vi "BaudDetect-Make Success Info.vi"(10 "Normal":bool, 11 "list":refnum<vi>) -> (3 "Info":string)   [LabVIEW 2011]
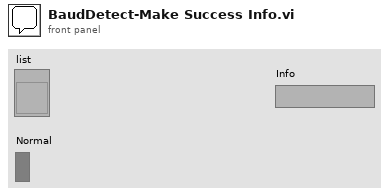
[diagram p1: front panel]
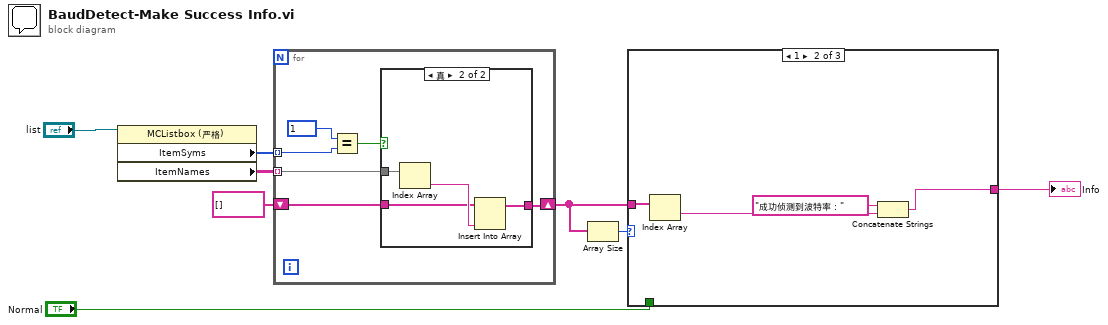
[diagram p0: block diagram]
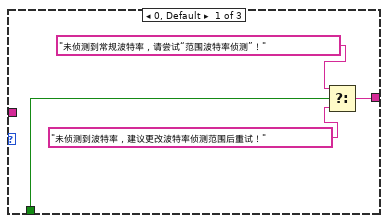
[diagram p2: hidden frame]
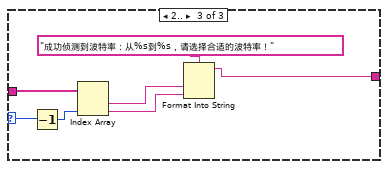
[diagram p3: hidden frame]
diagram:
  n1 = property class="MCListbox (严格)"(reference="list") -> ("ItemSyms"=w7:i32[], "ItemNames"=w6:string[][])  [unwired: 1 in, 2 out]
  n2 = for {
    tunnel: w7 -> [w14] mode=indexing
    tunnel: w6 -> [w11] mode=indexing
    shift-right: [w10] -> w3
    shift-left: string[] [] -> [w9]
    n3 = Equal?(x=1, y=w14) -> (x = y?=w12:bool)
    n4 = case shown="真" w12 {
      tunnel: w11 -> [_ w19]
      tunnel: [w15 w17] -> w10
      tunnel: w9 -> [w15 w16]
      frame False {
      }
      frame True {
        n5 = Index Array(array=w19) -> (element=w18:string)  [unwired: 1 in]
        n6 = Insert Into Array(array=w16, new element=w18) -> (w17:string[])  [unwired: 1 in]
      }
    }
  }
  n7 = Array Size(array=w3) -> (size(s)=w4:i32)
  n8 = case shown="1" w4 {
    selector: w4 -> [_ _ w33]
    tunnel: w3 -> [_ w27 w34]
    tunnel: "Normal" -> [w23 _ _]
    tunnel: [w20 w25 w28] -> w1
    frame 0, Default {
      n9 = Select(t="未侦测到常规波特率，请尝试“范围波特率侦测”！", s=w23, f="未侦测到波特率，建议更改波特率侦测范围后重试！") -> (s? t:f=w20:string)
    }
    frame 1 {
      n10 = Index Array(array=w27) -> (element=w26:string)  [unwired: 1 in]
      n11 = Concatenate Strings("成功侦测到波特率：" ("字符串"), w26) -> (w25:string)
    }
    frame 2.. {
      n12 = Decrement(x=w33) -> (x-1=w32:i32)
      n13 = Index Array(array=w34, index #2=w32) -> (element #1=w31:string, element #2=w30:string)  [unwired: 1 in]
      n14 = Format Into String(format string="成功侦测到波特率：从%s到%s，请选择合适的波特率！" ("格式字符串"), w31, w30) -> (resulting string=w28:string)  [unwired: 2 in, 1 out]
    }
  }
  "Info" <- w1
